vi "aft_xmpl_Simulate an Unknown System (Waveform).vi"(8 "error in (no error)":errorcluster, 9 "unknown system coefficients":dbl[](array[numeric])=[9.745429581298439e-18, 0.020461734458116075, 0.031830988618379075, 0.025008786559919588, -4.508492604200419e-17, -0.03215415414846812, -0.053051647697298455, -0.04501581580785527, 8.042442250270995e-17, 0.07502635967975894, 0.15915494309189543, 0.2250790790392766, 0.25, 0.2250790790392766, 0.15915494309189543, 0.07502635967975894, 8.042442250270995e-17, -0.04501581580785527, -0.053051647697298455, -0.03215415414846812, -4.508492604200419e-17, 0.025008786559919588, 0.031830988618379075, 0.020461734458116075, 9.745429581298439e-18], 10 "noise level":dbl=0.001, 11 "sampling info":cluster{"Fs":dbl, "#s":dbl}={"Fs"=1000.0, "#s"=1000.0} {"Fs" format="%.2p"}) -> (0 "error out":errorcluster, 1 "unknown system coefficients":dbl[](array[numeric]), 2 "response signal":waveform(dbl), 3 "stimulus signal":waveform(dbl))   [LabVIEW 2019]
doc: "Simulates the stimulus and response signals of an unknown system in block-by-block mode with waveform datatype. This VI uses a lowpass FIR filter to simulate the unknown system. The input or stimulus to the unknown system is Gaussian white noise. The output or response of the unknown system is the input signal passing through the FIR filter."
uses:
  <vilib>/measure/macond.llb/Continuous Waveform Convolution for 1 Chan.vi
  <vilib>/measure/NI_MABase.lvlib
  <vilib>/measure/NI_MAPro.lvlib
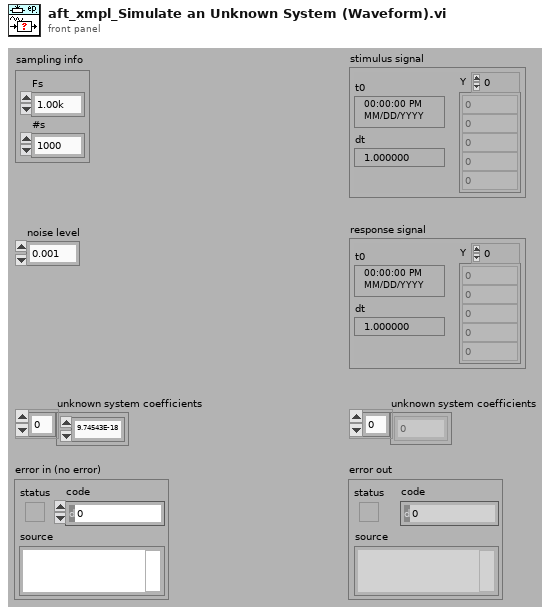
[diagram p1: front panel]
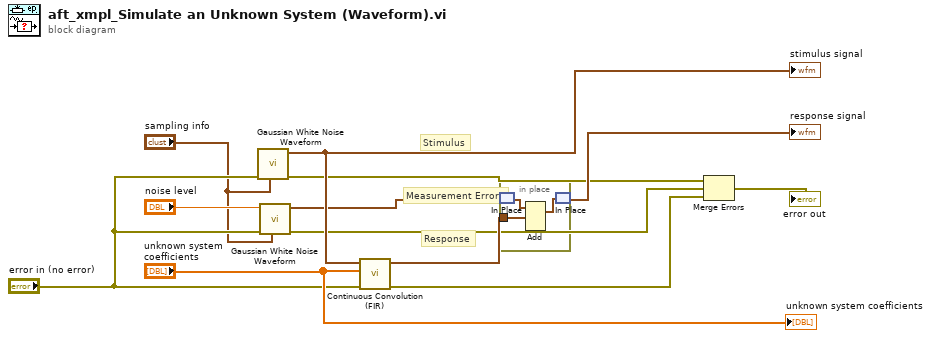
[diagram p0: block diagram]
diagram:
  # "Measurement Error"
  # "Stimulus"
  # "Response"
  n1 = call <vilib>:"Gaussian White Noise Waveform.vi"("sampling info"="sampling info", "error in (no error)"="error in (no error)") -> ("error out"=w5:errorcluster, "signal out"=w10:waveform(dbl))  [unwired: 3 in, 5 out]
  "stimulus signal" <- w10
  n2 = call <vilib>:"Gaussian White Noise Waveform.vi"("sampling info"="sampling info", "error in (no error)"="error in (no error)", "standard deviation"="noise level") -> ("error out"=w4:errorcluster, "signal out"=w9:waveform(dbl))  [unwired: 2 in, 5 out]
  n3 = call-poly <vilib>:"Continuous Convolution (FIR).vi"("error in (no error)"="error in (no error)", "kernel"="unknown system coefficients", "signal in"=w10) -> ("error out"=w3:errorcluster, "signal out"=w8:waveform(dbl))  [unwired: 3 in, 4 out]
  n4 = in-place {
    in-place-border: w8 -> [w13]
    n5 = in-place-match #1(w9) -> (w14:waveform(dbl))
    n6 = Add(1:w13, 2:w14) -> (0:w15:waveform(dbl))  [unwired: 1 in, 1 out]
    n7 = in-place-match #1(w15) -> (→"response signal":waveform(dbl))
  }
  n8 = Merge Errors(w5, w4, w3) -> (→"error out":errorcluster)
  "unknown system coefficients" <- "unknown system coefficients"
